vi "Find peaks.vi"(7 "Frequency Axis Scale Factor":dbl format="%#_13g", 10 "FFT (single frame)":dbl[](array[numeric])) -> (1 "Peak Magnitudes":dbl[](array[numeric]), 2 "Peaks Frequencies":dbl[](array[numeric]))   [LabVIEW 2014, in "Melody Extraction.lvlib"]
uses:
  Melody Extraction.lvlib
  <vilib>/Analysis/NI_AAL_SigProc.lvlib
panel:
  out "Waveform Graph 3":dbl[](graph)
  out "Waveform Graph 2":dbl[](graph)
  out "Waveform Graph":dbl[](graph)
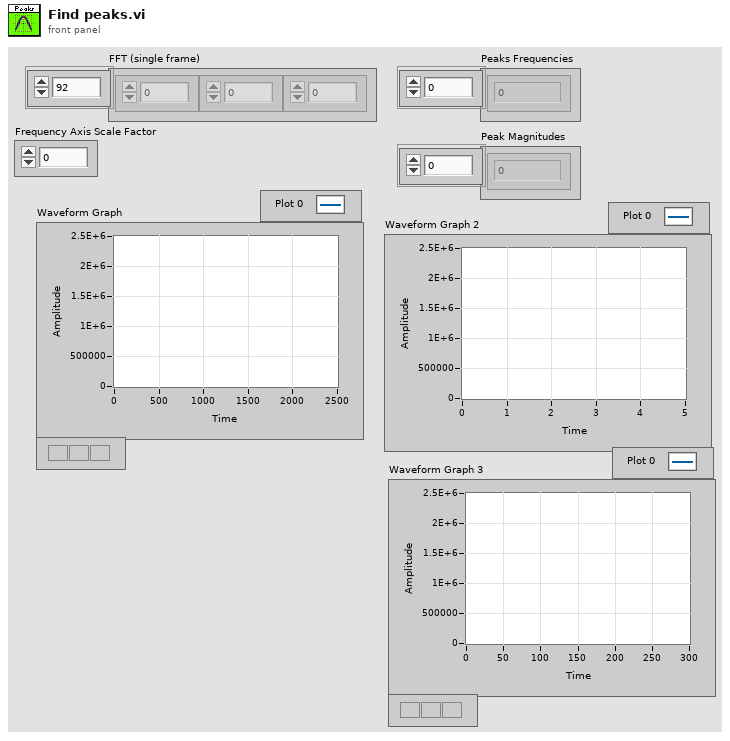
[diagram p1: front panel]
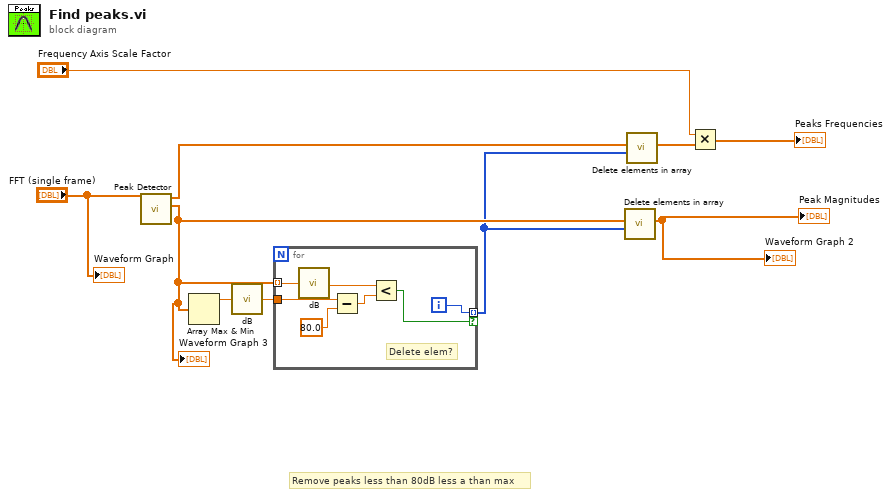
[diagram p0: block diagram]
diagram:
  # "Remove peaks less than 80dB less a than max"
  n1 = call <vilib>:"Peak Detector.vi"("X"="FFT (single frame)") -> ("Amplitudes"=w4:dbl[], "Locations"=w5:dbl[])  [unwired: 6 in, 3 out]
  "Waveform Graph 3" <- w4
  n2 = Array Max & Min(array=w4) -> (max value=w7:dbl)  [unwired: 3 out]
  n3 = call "dB.vi"("V"=w7) -> ("dB"=w6:dbl)
  n4 = for {
    tunnel: w4 -> [w17] mode=indexing
    tunnel: [w13] -> w3 mode=indexing if=w12
    tunnel: w6 -> [w11]
    i -> [w13]
    # "Delete elem?"
    n5 = call "dB.vi"("V"=w17) -> ("dB"=w14:dbl)
    n6 = Subtract(x=w11, y=80.0) -> (x-y=w15:dbl)
    n7 = Less?(x=w14, y=w15) -> (x < y?=w12:bool)
  }
  n8 = call "Delete elements in array.vi"("Elements to Delete"=w3, "Input Array"=w4) -> ("Output Array"=→"Peak Magnitudes" →"Waveform Graph 2":dbl[])  [unwired: 9 in]
  n9 = call "Delete elements in array.vi"("Elements to Delete"=w3, "Input Array"=w5) -> ("Output Array"=w2:dbl[])  [unwired: 9 in]
  n10 = Multiply(x="Frequency Axis Scale Factor", y=w2) -> (x*y=→"Peaks Frequencies":dbl[])
  "Waveform Graph" <- "FFT (single frame)"
